vi "tcp close.vi"(6 "length":i32, 8 "error in":errorcluster, 9 "Address":i32, 10 "Write Data":sgl[](array[numeric])=[1.0, 1.0, 1.0, 1.0, 1.0, 1.0, 1.0, 1.0, 1.0, 1.0, 1.0, 1.0, 1.0, 1.0, 1.0, 100.0, 100.0, 100.0, 100.0, 100.0, 0.0, 100.0, 100.0, 100.0], 11 "connection ID IN":refnum<k5>) -> (0 "error out":errorcluster, 3 "connection ID out":refnum<k5>)   [LabVIEW 2015]
panel:
  out "subarray":sgl[](array[numeric])
  out "substring":string
  out "data out":string
  out "concatenated string":string
  out "Total Characters":i32
  out "Total Array":i32
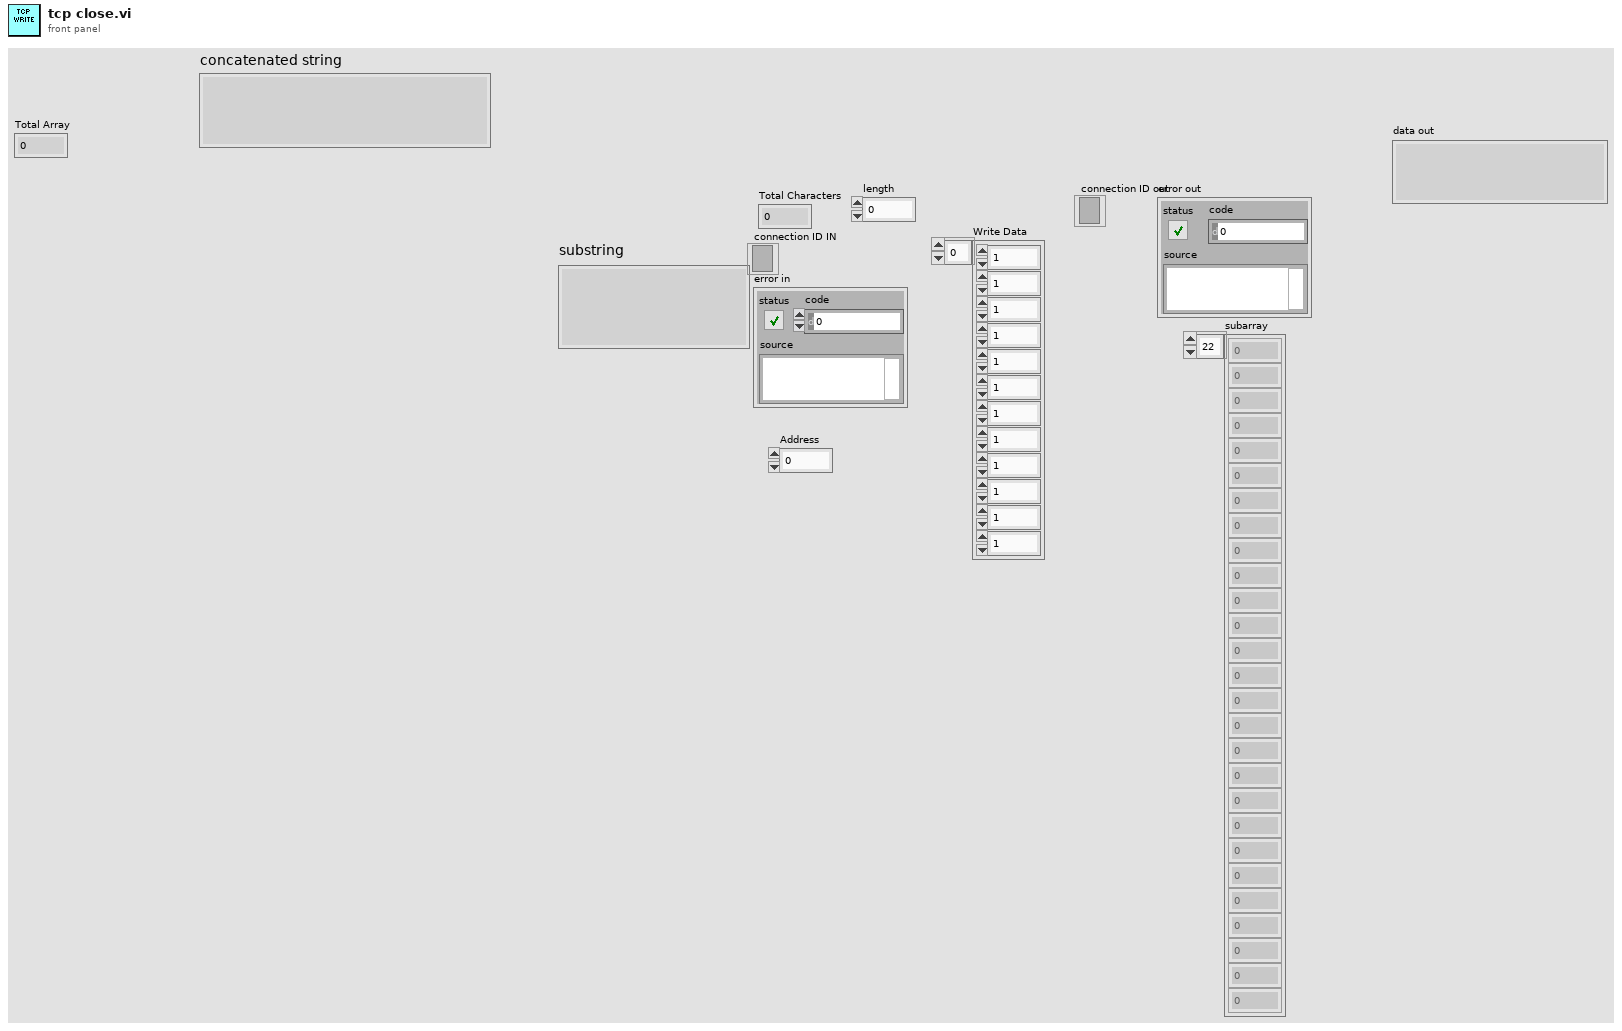
[diagram p1: front panel]
types:
  T1 = enum16{"Standard", "Buffered", "CRLF", "Immediate"}
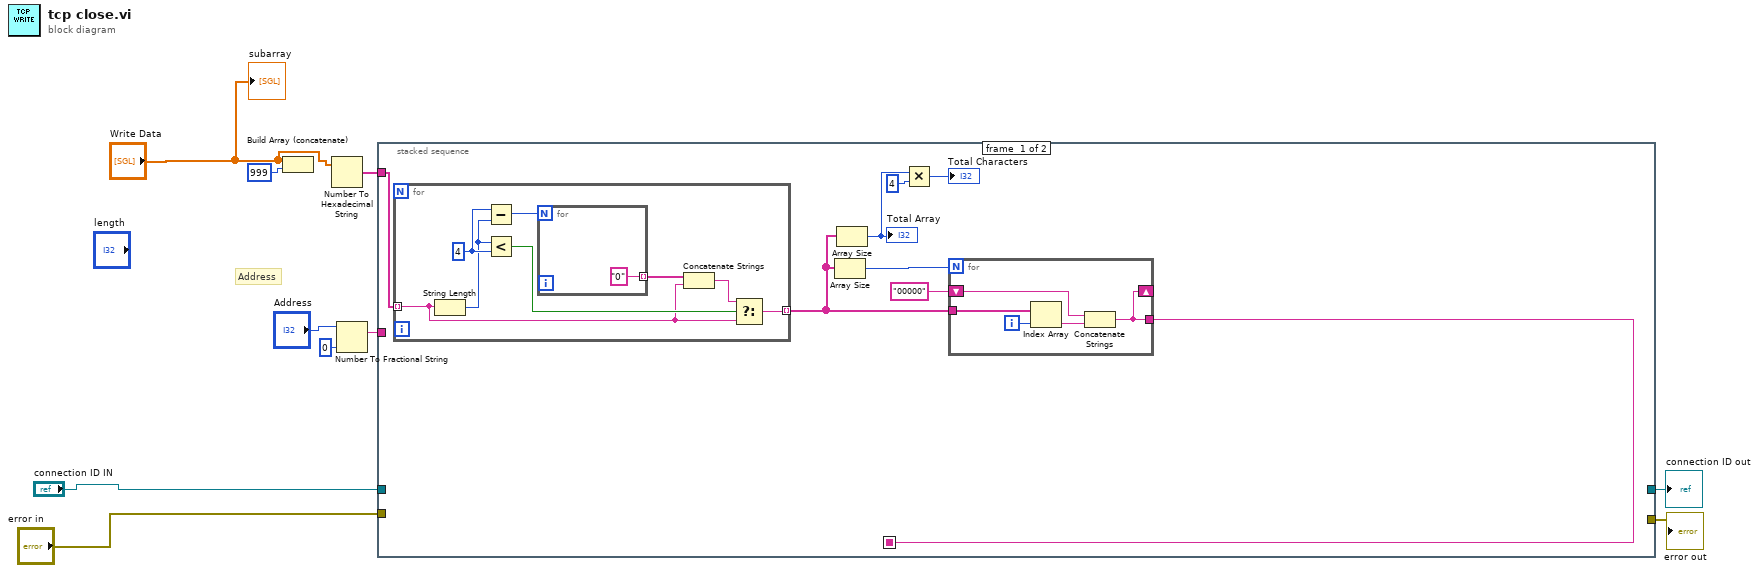
[diagram p0: block diagram]
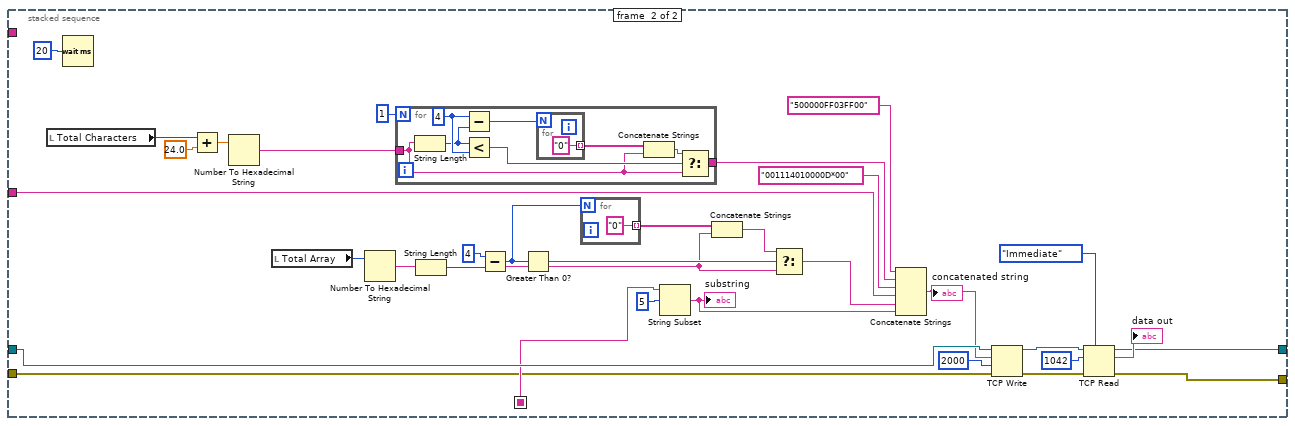
[diagram p2: hidden frame]
diagram:
  # "Address"
  n1 = Build Array (concatenate)("Write Data", 999) -> ()  [unwired: 1 out]
  n2 = Number To Hexadecimal String(2:"Write Data") -> (0:w9:string[])  [unwired: 1 in]
  n3 = Number To Fractional String(number="Address", precision (6)=i16 0) -> (F-format string=w4:string)  [unwired: 2 in]
  n4 = stacked-sequence {
    seq-local: [w17 _] -> [_ w63]
    tunnel: "connection ID IN" -> [_ w65]
    tunnel: w9 -> [w11 _]
    tunnel: "error in" -> [_ w37]
    tunnel: [_ w36] -> w8
    tunnel: [_ w35] -> w7
    tunnel: w4 -> [_ w34]
    frame #0 {
      n5 = for {
        tunnel: w11 -> [w21] mode=indexing
        tunnel: [w19] -> w12 mode=indexing
        w25 = 4 ("y")
        n6 = String Length(string=w21) -> (length=w24:i32)
        n7 = Subtract(x=w25, y=w24) -> (x-y=w23:i32)
        n8 = Less?(x=w24, y=w25) -> (x < y?=w26:bool)
        n9 = for {
          N: w23 -> [_]
          tunnel: ["0"] -> w22 mode=indexing
        }
        n10 = Concatenate Strings(w22, w21) -> (w20:string)
        n11 = Select(t=w20, s=w26, f=w21) -> (s? t:f=w19:string)
      }
      n12 = Array Size(array=w12) -> (size(s)=w16:i32)
      n13 = Array Size(array=w12) -> (size(s)=w13:i32)
      "Total Array" <- w13
      n14 = Multiply(x=w13, y=4) -> (x*y=→"Total Characters":i32)
      n15 = for {
        N: w16 -> [_]
        shift-right: [w30] -> _
        shift-left: "00000" -> [w29]
        tunnel: [w30] -> w17
        tunnel: w12 -> [w28]
        i -> [w32]
        n16 = Index Array(array=w28, index=w32) -> (element=w31:string)
        n17 = Concatenate Strings(w29, w31) -> (w30:string)
      }
    }
    frame #1 {
      n18 = local read "Total Characters"() -> (w39:i32)
      n19 = Wait (ms)(milliseconds to wait=u32 20) -> ()  [unwired: 1 out]
      n20 = Add(x=w39, y=24.0) -> (x+y=w51:dbl)
      n21 = Number To Hexadecimal String(2:w51) -> (0:w52:string)  [unwired: 1 in]
      n22 = local read "Total Array"() -> (w38:i32)
      n23 = Number To Hexadecimal String(2:w38) -> (0:w57:string)  [unwired: 1 in]
      n24 = for {
        N: 1 -> [_]
        tunnel: w52 -> [w68]
        tunnel: [w66] -> w42
        w72 = 4 ("y")
        n25 = String Length(string=w68) -> (length=w71:i32)
        n26 = Subtract(x=w72, y=w71) -> (x-y=w70:i32)
        n27 = Less?(x=w71, y=w72) -> (x < y?=w73:bool)
        n28 = for {
          N: w70 -> [_]
          tunnel: ["0"] -> w69 mode=indexing
        }
        n29 = Concatenate Strings(w69, w68) -> (w67:string)
        n30 = Select(t=w67, s=w73, f=w68) -> (s? t:f=w66:string)
      }
      n31 = String Length(string=w57) -> (length=w61:i32)
      n32 = Subtract(x=4, y=w61) -> (x-y=w33:i32)
      n33 = Greater Than 0?(x=w33) -> (x > 0?=w59:bool)
      n34 = for {
        N: w33 -> [_]
        tunnel: ["0"] -> w47 mode=indexing
      }
      n35 = String Subset(string=w63, offset (0)=5) -> (substring=w48:string)  [unwired: 1 in]
      "substring" <- w48
      n36 = Concatenate Strings(w47, w57) -> (w58:string)
      n37 = Select(t=w58, s=w59, f=w57) -> (s? t:f=w41:string)
      n38 = Concatenate Strings("500000FF03FF00" ("data in"), w42, "001114010000D*00" ("data in"), w34, w41, w48) -> (w53:string)
      "concatenated string" <- w53
      n39 = TCP Write(connection ID=w65, data in=w53, error in (no error)=w37, 9:2000 ("timeout ms (25000)")) -> (connection ID out=w56:refnum<k5>, error out=w55:errorcluster)  [unwired: 1 out]
      n40 = TCP Read(connection ID=w56, bytes to read=1042, error in (no error)=w55, 7:T1."Immediate" ("mode (standard)")) -> (connection ID out=w36:refnum<k5>, data out=→"data out":string, error out=w35:errorcluster)  [unwired: 1 in]
    }
  }
  "connection ID out" <- w8
  "error out" <- w7
  "subarray" <- "Write Data"
